vi "BRig_Host_dataRunState__entryDelete.vi"() -> ()   [LabVIEW 2014]
panel:
  out "output_arrTrials":u16[](array[numeric])
  out "output_arrTrials_length":i32
  out "output_arrTrials":bool
  out "output_dataPlot":u16[][](array[numeric])
  out "output_idx":i32[](array[numeric])
  in  "input_nTrial":u16
  in  "input_idx":i32[](array[numeric])
  in  "input_dataTS":u16[][](array[numeric])
  in  "input_dataPlot":u16[][](array[numeric])
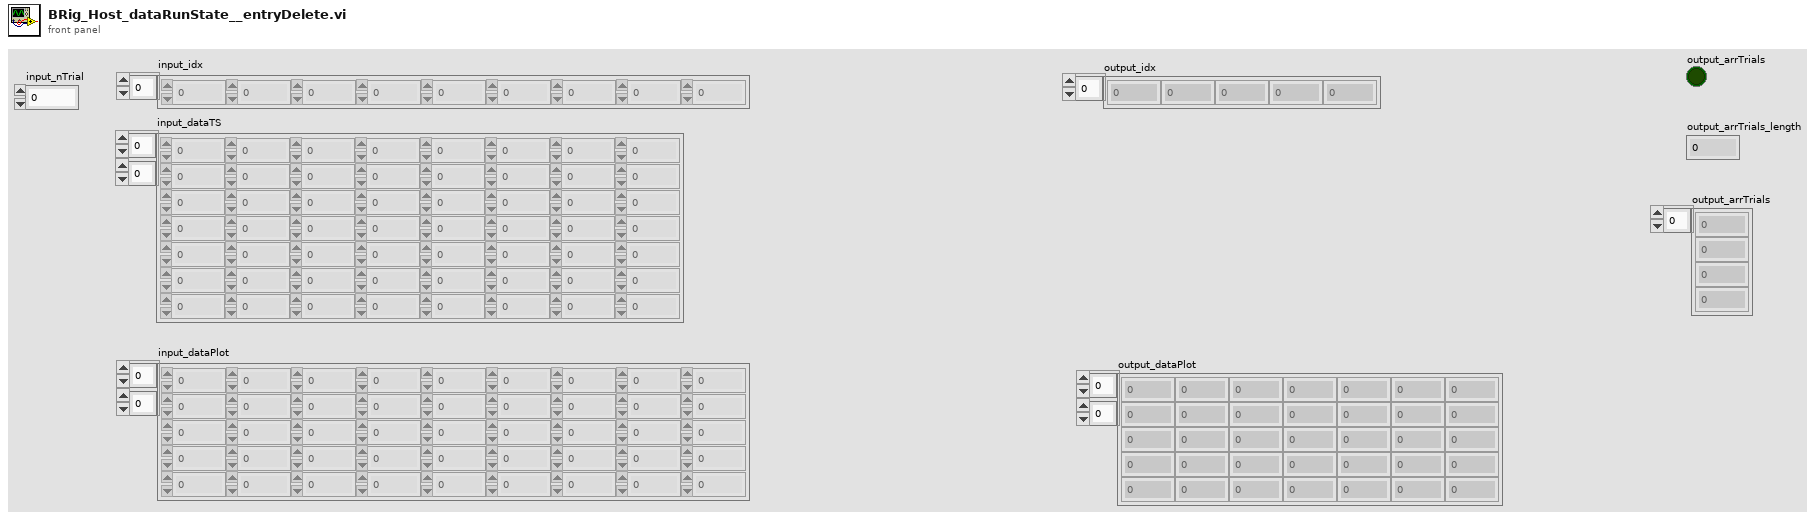
[diagram p1: front panel]
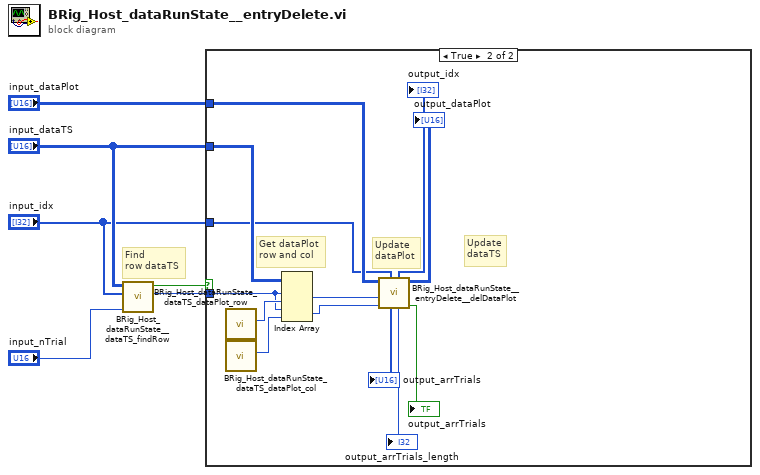
[diagram p0: block diagram]
diagram:
  # "Find\nrow dataTS"
  n1 = call "BRig_Host_dataRunState__dataTS_findRow.vi"("input_nTrial"="input_nTrial", "input_idx"="input_idx", "input_dataTS"="input_dataTS") -> ("output_row_dataTS"=w3:i32, "output_I_row_dataTS"=w4:bool)  [unwired: 7 in]
  n2 = case shown="True" w4 {
    tunnel: "input_dataTS" -> [_ w19]
    tunnel: w3 -> [_ w17]
    tunnel: "input_dataPlot" -> [_ w15]
    tunnel: "input_idx" -> [_ w8]
    frame False {
    }
    frame True {
      # "Update\ndataTS"
      # "Update\ndataPlot"
      # "Get dataPlot\nrow and col"
      n3 = call "BRig_Host_dataRunState_dataTS_dataPlot_row.vi"() -> ("output_idx_dataTS_dataPlot_row"=w18:i32)  [unwired: 11 in]
      n4 = call "BRig_Host_dataRunState_dataTS_dataPlot_col.vi"() -> ("output_idx_dataTS_dataPlot_col"=w16:i32)  [unwired: 11 in]
      n5 = Index Array(array=w19, index (row) #1=w17, index (col) #1=w18, index (row) #2=w17, index (col) #2=w16) -> (element #1=w14:u16, element #2=w13:u16)
      n6 = call "BRig_Host_dataRunState__entryDelete__delDataPlot.vi"("input_idx"=w8, "input_col_dataPlot"=w13, "input_row_dataPlot"=w14, "input_dataPlot"=w15) -> (0:"output_arrTrials"=→"output_arrTrials":bool, "output_dataPlot"=→"output_dataPlot":u16[][], "output_arrTrials_length"=→"output_arrTrials_length":i32, "output_idx"=→"output_idx":i32[], 6:"output_arrTrials"=→"output_arrTrials":i32[])  [unwired: 3 in]
    }
  }
